vi "PV Change Pressure.vi"(1 "Pressure String":string) -> (0 "Change Pressure String":string)   [LabVIEW 2015, in "Pfeiffer Vacuum.lvlib"]
uses:
  Pfeiffer Vacuum.lvlib
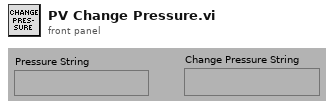
[diagram p1: front panel]
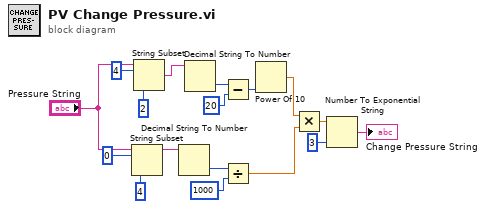
[diagram p0: block diagram]
diagram:
  n1 = String Subset(string="Pressure String", offset (0)=0, length (rest)=4) -> (substring=w8:string)
  n2 = String Subset(string="Pressure String", offset (0)=4, length (rest)=2) -> (substring=w9:string)
  n3 = Decimal String To Number(string=w8) -> (number=w12:i32)  [unwired: 2 in, 1 out]
  n4 = Decimal String To Number(string=w9) -> (number=w13:i32)  [unwired: 2 in, 1 out]
  n5 = Subtract(x=w13, y=20) -> (x-y=w14:i32)
  n6 = Divide(x=w12, y=1000) -> (x/y=w15:dbl)
  n7 = Power Of 10(x=w14) -> (10^x=w16:dbl)
  n8 = Multiply(x=w16, y=w15) -> (x*y=w3:dbl)
  n9 = Number To Exponential String(number=w3, precision (6)=i16 3 ("Genauigkeit (6)")) -> (E-format string=→"Change Pressure String":string)  [unwired: 2 in]
